vi "Image_Processing_Queue_2.0.vi"(5 "Data":T1={"Camera 1"={"Camera1"="", "Cam 1"=FALSE, "CAM1 Model"=enum."a2A5328-15ucBAS", "Cam1 ID"=0}, "Camera 2"={"Camera2"="", "Cam 2"=FALSE, "CAM2 Model"=enum."a2A5328-15ucBAS", "Cam2 ID"=0}, "Image"={"Camera1_Img"=refnum, "Camera2_Img"=refnum, "Img1_Orig_Disp"=refnum, "Img2_Orig_Disp"=refnum, "Img1_Orig_RGB"=refnum, "Img2_Orig_RGB"=refnum, "Blue_Plane_Extract"=refnum, "Subtracted_Plane"=refnum, "Img1_Binary"=refnum, "Img2_Binary"=refnum, "Crop_Mask"=refnum, "Img1_Save"=refnum, "Img2_Save"=refnum, "Img1_Cali_Full"=refnum, "Img2_Cali_Full"=refnum, "Img1_Cali_Detect"=refnum, "Img2_Cali_Detect"=refnum}, "Ques"={"Cam 1 queue"=refnum, "Cam 2 queue"=refnum, "Cam 1 - save queue"=refnum, "Cam 2 - save queue"=refnum, "Image Process Queue Size"=500, "Image Save Queue Size"=500, "Overload threshold"=500, "Max large object threshold"=0}, "Arduino SRS"={"Pinch-valve"="", "Actuator"=FALSE, "Arduino Uno"="", "Valve state"=enum."Open"}, "Pump"={"Port"="", "Connection"=FALSE, "Flush Size"=0, "Command"="", "Pump Size"=enum."Large", "Pump"="", "Ready"=FALSE}, "Camera settings"={"Detection settings"={"Sample size threshold"=500, "Detection Region %"=30.0, "Timeout Sample"=200}, "Lens/camera settings"={"Aperture"=enum."Item 0", "Legacy Cam Attributes"=FALSE, "Max Framerate"=100, "Exposure Time"=1000.0, "Framerate"=15}, "Crop settings"={"Cam1"={"Rectangle 1"={"Left"=0, "Top"=0, "Right"=0, "Bottom"=0, "Rotation"=0.0}, "Camera Orientation 1"="", "Pixel to mm 1"=0.0}, "Cam2"={"Rectangle 2"={"Left"=0, "Top"=0, "Right"=0, "Bottom"=0, "Rotation"=0.0}, "Camera Orientation 2"="", "Pixel to mm 2"=0.0}}}, "Arduino ISS"={"Mega F3"="", "Phase3"=FALSE, "Barcode"="", "Sorting sys."=FALSE, "Initial size"=0.0, "Size Interval"=0.0, "Mun. of containers"=0.0, "Container nr."=0.0, "Arduino Mega"="", "Attempts"=0.0}, "Img_Capt"=FALSE, "Empty_Refill"=FALSE, "I don't think is in use"={"Light intensity"=100}, "Extended setup"={"Location"="Station", "Latitude"="Station", "Longitude"="Station", "Determiner"="Station", "Sex"="Station", "Station"="", "Collection date"=""}, "Main interface"={"Sample Name"="Test Sample", "Operator"="JFR", "Species Name"="", "Other Notes"=""}, "Tap1"=0, "SystemVersion"=0, "System Serial"="", "Exit"=FALSE, "Kuvette Full"=FALSE, "Core JKI"={"Current VI Reference"=refnum, "Close Panel on Exit?"=FALSE}, "Calibration"={"Calibration 1"=path "C:/Users/au540322/Desktop/IHS_Project/images/Debris/Debris_0/Debris_0_2019_06_01-23-32-49-686.PNG", "Calibration 2"=path "C:/Users/au540322/Desktop/IHS_Project/images/Debris/Debris_0/Debris_0_2019_06_01-23-32-49-686.PNG", "Detect 1"=path "C:/Users/au540322/Desktop/IHS_Project/images/Debris/Debris_0/Debris_0_2019_06_01-23-32-49-686.PNG", "Detect 2"=path "C:/Users/au540322/Desktop/IHS_Project/images/Debris/Debris_0/Debris_0_2019_06_01-23-32-49-686.PNG"}, "Auto Flush"=FALSE, "Status History"="", "Timestamp Start"=""} {"SystemVersion" items=["Standard", "XL"]; "Tap1" items=["Session Data", "Extended Setup", "Buffer", "Camera", "Dispenser", "Stats", "Connections"]; "I don't think is in use"."Light intensity" scale=0.0..100.0; "Camera settings"."Crop settings"."Cam2"."Rectangle 2"."Rotation" format="%.2f"; "Camera settings"."Crop settings"."Cam2"."Rectangle 2"."Left" scale=0.0..1024.0; "Camera settings"."Crop settings"."Cam2"."Rectangle 2"."Right" scale=0.0..1024.0; "Camera settings"."Crop settings"."Cam1"."Rectangle 1"."Rotation" format="%.2f"; "Camera settings"."Crop settings"."Cam1"."Rectangle 1"."Left" scale=0.0..1024.0; "Camera settings"."Crop settings"."Cam1"."Rectangle 1"."Right" scale=0.0..1024.0; "Camera settings"."Lens/camera settings"."Framerate" min=1; "Camera settings"."Lens/camera settings"."Max Framerate" min=1; "Camera settings"."Detection settings"."Sample size threshold" min=1; "Pump"."Flush Size" min=0 max=6000 step=100; "Ques"."Overload threshold" min=1; "Ques"."Image Save Queue Size" min=1; "Ques"."Image Process Queue Size" min=1}) -> (10 "Status":T5, 11 "Detection error":errorcluster, 12 "Process queue":T6, 13 "Last Image?":bool, 14 "Object1":T3, 15 "Object2":T3, 16 "Image 1":T3, 17 "Image 2":T3, 18 "Binary 1":T3, 19 "Binary 2":T3)   [LabVIEW 2024]
doc: "Saves every 6th image in a sub folder in the current directory (specified from Sample Name). When a true is sent to Sample+1 a new subfolder is created with incremental numbering.\nExample of folders: \n../images/Sample_Name/Sample_Name1\n../images/Sample_Name/Sample_Name2"
uses:
  <vilib>/vision/Image Controls.llb/IMAQ Image.ctl
  <extravilib>/ChannelInstances/Tag-c(bool,bool)/))Channel.ctl
  controls/Data_JKI.ctl
  <vilib>/userDefined/High Color/IMAQdx.ctl
  Camera_ID.ctl
  <extravilib>/ChannelInstances/Tag-c(bool,bool)/Write With Abort.vi
  <extravilib>/ChannelInstances/Tag-c(bool,bool)/Endpoint.vi
  <extravilib>/ChannelInstances/Tag-c(bool,bool).lvlib
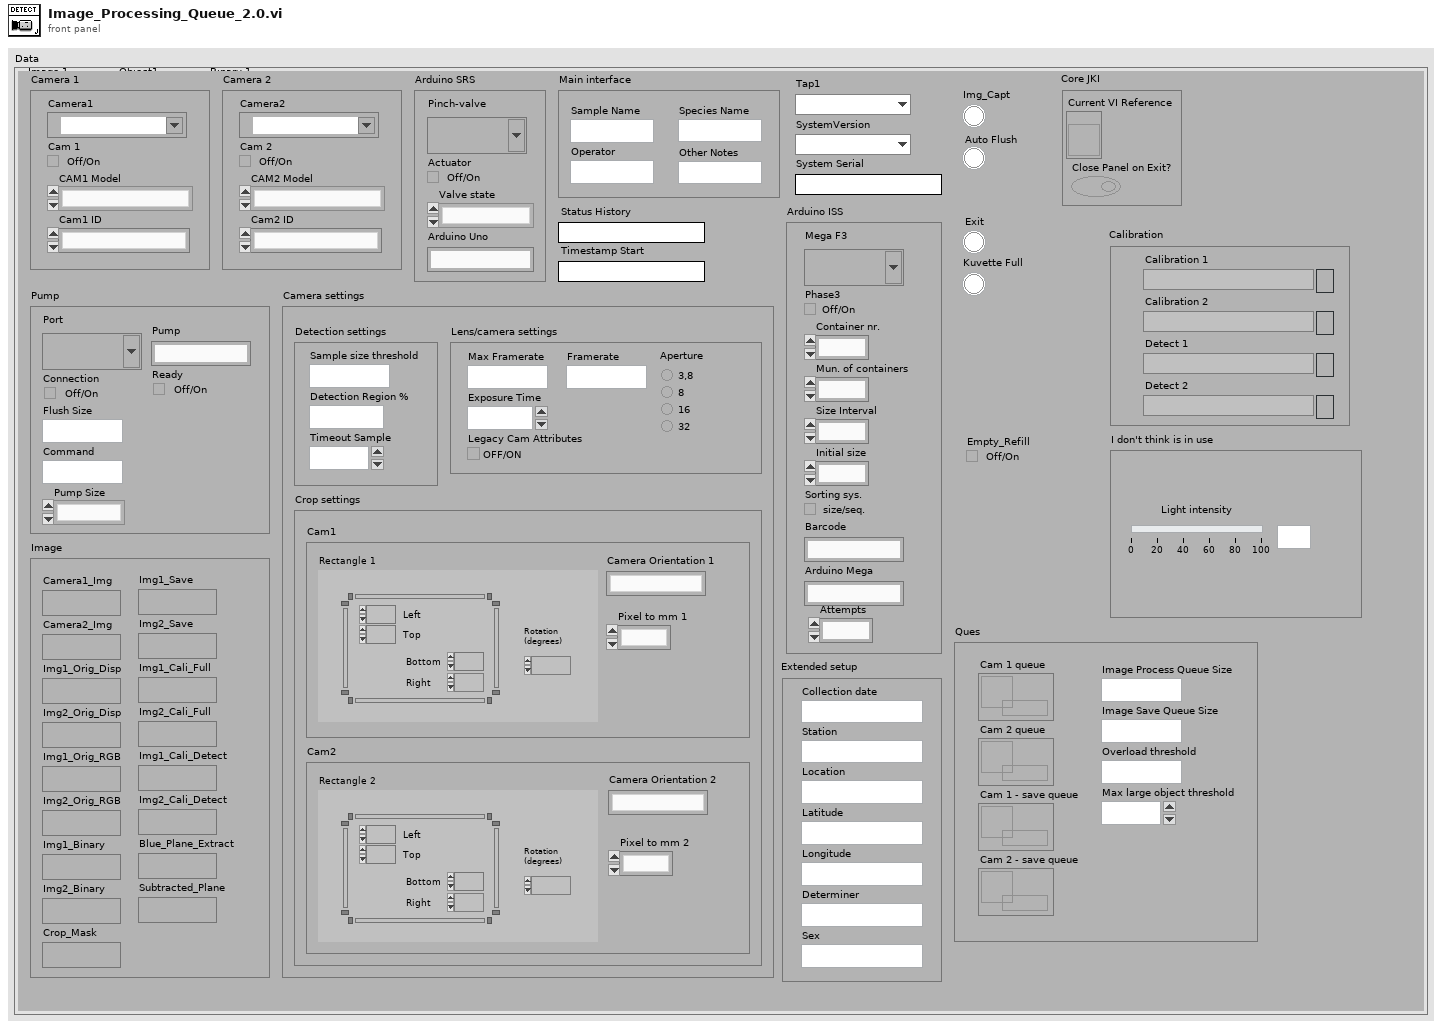
[diagram p1: front panel]
types:
  T1 = typedef "Data_JKI.ctl" = cluster{"Camera 1":cluster{"Camera1":T2, "Cam 1":bool, "CAM1 Model":enum16{"a2A5328-15ucBAS", "acA1920-155uc"}, "Cam1 ID":i32}, "Camera 2":cluster{"Camera2":T2, "Cam 2":bool, "CAM2 Model":enum16{"a2A5328-15ucBAS", "acA1920-155uc"}, "Cam2 ID":i32}, "Image":cluster{"Camera1_Img":T3, "Camera2_Img":T3, "Img1_Orig_Disp":T3, "Img2_Orig_Disp":T3, "Img1_Orig_RGB":T3, "Img2_Orig_RGB":T3, "Blue_Plane_Extract":T3, "Subtracted_Plane":T3, "Img1_Binary":T3, "Img2_Binary":T3, "Crop_Mask":T3, "Img1_Save":T3, "Img2_Save":T3, "Img1_Cali_Full":T3, "Img2_Cali_Full":T3, "Img1_Cali_Detect":T3, "Img2_Cali_Detect":T3}, "Ques":cluster{"Cam 1 queue":refnum<queue>, "Cam 2 queue":refnum<queue>, "Cam 1 - save queue":refnum<queue>, "Cam 2 - save queue":refnum<queue>, "Image Process Queue Size":i32, "Image Save Queue Size":i32, "Overload threshold":i32, "Max large object threshold":i32}, "Arduino SRS":cluster{"Pinch-valve":refnum<visa-resource-name>, "Actuator":bool, "Arduino Uno":string, "Valve state":enum16{"Standby", "Close", "Open"}}, "Pump":cluster{"Port":refnum<visa-resource-name>, "Connection":bool, "Flush Size":i32, "Command":string, "Pump Size":enum16{"None", "Small", "Large"}, "Pump":string, "Ready":bool}, "Camera settings":cluster{"Detection settings":cluster{"Sample size threshold":i32, "Detection Region %":dbl, "Timeout Sample":i32}, "Lens/camera settings":cluster{"Aperture":enum32{"Item 0", "Item 1", "Item 2", "Item 3"}, "Legacy Cam Attributes":bool, "Max Framerate":i32, "Exposure Time":dbl, "Framerate":i32}, "Crop settings":cluster{"Cam1":cluster{"Rectangle 1":T4, "Camera Orientation 1":string, "Pixel to mm 1":dbl}, "Cam2":cluster{"Rectangle 2":T4, "Camera Orientation 2":string, "Pixel to mm 2":dbl}}}, "Arduino ISS":cluster{"Mega F3":refnum<visa-resource-name>, "Phase3":bool, "Barcode":string, "Sorting sys.":bool, "Initial size":dbl, "Size Interval":dbl, "Mun. of containers":dbl, "Container nr.":dbl, "Arduino Mega":string, "Attempts":dbl}, "Img_Capt":bool, "Empty_Refill":bool, "I don't think is in use":cluster{"Light intensity":i32}, "Extended setup":cluster{"Location":string, "Latitude":string, "Longitude":string, "Determiner":string, "Sex":string, "Station":string, "Collection date":string}, "Main interface":cluster{"Sample Name":string, "Operator":string, "Species Name":string, "Other Notes":string}, "Tap1":u16, "SystemVersion":u16, "System Serial":string, "Exit":bool, "Kuvette Full":bool, "Core JKI":cluster{"Current VI Reference":refnum<vi>, "Close Panel on Exit?":bool}, "Calibration":cluster{"Calibration 1":path, "Calibration 2":path, "Detect 1":path, "Detect 2":path}, "Auto Flush":bool, "Status History":string, "Timestamp Start":string}
  T2 = typedef "IMAQdx.ctl" = refnum<k21>
  T3 = typedef "IMAQ Image.ctl" = refnum<image>
  T4 = typedef "IMAQ Rectangle" = cluster{"Left":i32, "Top":i32, "Right":i32, "Bottom":i32, "Rotation":dbl}
  T5 = typedef "Tag-c(bool,bool).lvlib/))Channel.ctl" = refnum<queue>
  T6 = cluster{"# elements in queue":i32, "# elements in queue":i32}
  T7 = typedef "Camera_ID.ctl" = enum16{"Camera 1", "Camera 2"}
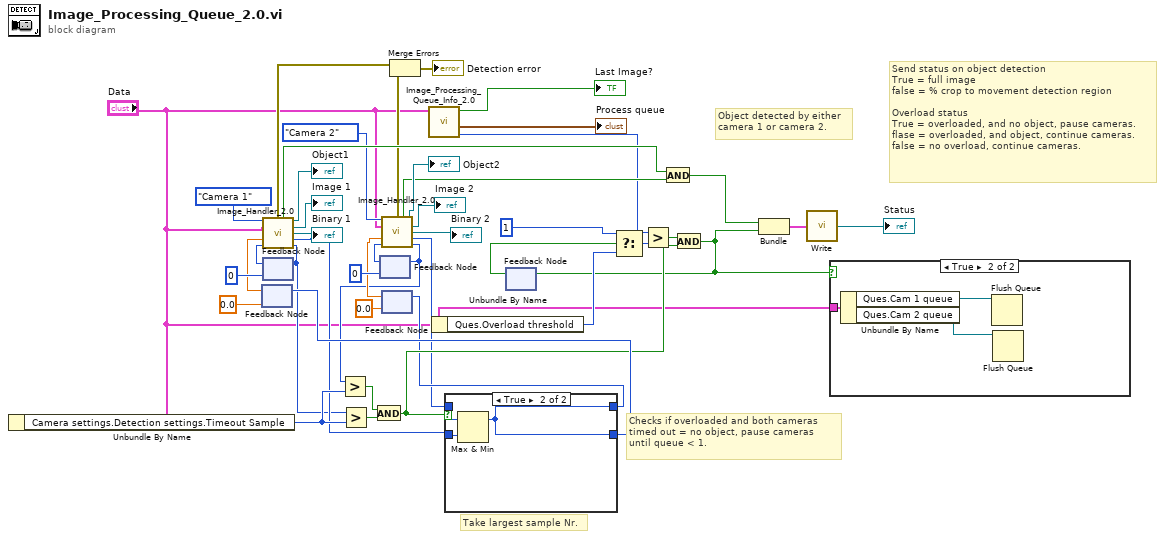
[diagram p0: block diagram]
diagram:
  # "Take largest sample Nr."
  # "Send status on object detection\nTrue = full image\nfalse = % crop to movement detection region\n\nOverload status\nTrue = overloaded, and no object, pause cameras.\nflase = overloaded, and object, continue cameras.\nfalse = no overload, continue cameras."
  # "Object detected by either\ncamera 1 or camera 2."
  # "Checks if overloaded and both cameras \ntimed out = no object, pause cameras \nuntil queue < 1."
  n1 = Unbundle By Name("Data") -> ("Camera settings.Detection settings.Timeout Sample"=w39:i32)
  n2 = feedback #1(0.0 ("Sample nr")) -> (w16:dbl)
  n3 = feedback #2(0 ("Timeout out")) -> (w17:i32)
  n4 = call "Image_Handler_2.0.vi"("Camera"=Camera_ID."Camera 1", "Data"="Data", "Prev. sample"=w16, "Timeout in"=w17) -> ("Detection error"=w24:errorcluster, "Object"=w23:bool, "Detected object"=→"Object1":T3, "Image Out"=→"Image 1":T3, "Binary"=→"Binary 1":T3, "Sample nr"=w20:i32, "Timeout out"=w18:i32)  [unwired: 5 in]
  n5 = feedback-in #2(w18) -> ()
  n6 = Greater?(x=w18, y=w39) -> (0:w40:bool)
  n7 = feedback #3(0 ("Timeout out")) -> (w13:i32)
  n8 = feedback #4(0.0 ("Sample nr")) -> (w12:dbl)
  n9 = call "Image_Handler_2.0.vi"("Camera"=Camera_ID."Camera 2", "Data"="Data", "Prev. sample"=w12, "Timeout in"=w13) -> ("Detection error"=w5:errorcluster, "Object"=w6:bool, "Detected object"=→"Object2":T3, "Image Out"=→"Image 2":T3, "Binary"=→"Binary 2":T3, "Sample nr"=w10:i32, "Timeout out"=w11:i32)  [unwired: 5 in]
  n10 = Greater?(x=w11, y=w39) -> (0:w38:bool)
  n11 = And(x=w38, y=w40) -> (x .and. y?=w27:bool)
  n12 = feedback-in #3(w11) -> ()
  n13 = Merge Errors(w24, w5) -> (→"Detection error":errorcluster)
  n14 = call "Image_Processing_Queue_Info_2.0.vi"("Data"="Data") -> ("Max Queue Size"=w1:i32, "Queue data"=→"Process queue":T6, "Last Image?"=→"Last Image?":bool)  [unwired: 4 in]
  n15 = Unbundle By Name("Data") -> ("Ques.Overload threshold"=w33:i32)
  n16 = case shown="True" w27 {
    tunnel: w10 -> [w45 w49]
    tunnel: w20 -> [w46 w48]
    tunnel: [w46 w47] -> w28
    tunnel: [w45 w47] -> w26
    frame False {
    }
    frame True {
      n17 = Max & Min(x=w49, y=w48) -> (max(x,y)=w47:i32)  [unwired: 1 out]
    }
  }
  n18 = feedback-in #1(w28) -> ()
  n19 = feedback-in #4(w26) -> ()
  n20 = feedback #5() -> (w35:bool)  [unwired: 1 in]
  n21 = Select(t=1 ("y"), s=w35, f=w33) -> (s? t:f=w34:i32)
  n22 = Greater?(x=w1, y=w34) -> (0:w37:bool)
  n23 = And(x=w23, y=w6) -> (x .and. y?=w32:bool)
  n24 = And(x=w37, y=w27) -> (x .and. y?=w25:bool)
  n25 = feedback-in #5(w25) -> ()
  n26 = Bundle(w32, w25) -> (w31:cluster{bool, bool})  [unwired: 1 in]
  n27 = call <extravilib>:"Write.vi"("element"=w31) -> ("channel"=→"Status":T5)  [unwired: 1 out]
  n28 = case shown="True" w25 {
    tunnel: "Data" -> [_ w52]
    frame False {
    }
    frame True {
      n29 = Unbundle By Name(w52) -> ("Ques.Cam 1 queue"=w51:refnum<queue>, "Ques.Cam 2 queue"=w50:refnum<queue>)
      n30 = Flush Queue(queue=w51) -> ()  [unwired: 1 in, 3 out]
      n31 = Flush Queue(queue=w50) -> ()  [unwired: 1 in, 3 out]
    }
  }
